vi "DIO_in.vi"(9 "Digital Pin":string(combo)="Y9", 11 "Data In":T1) -> (3 "Data Out":T1={"Port"="", "All Code"="Hi"})   [LabVIEW 2016]
uses:
  uPythonX/PythonData.ctl
  uPythonX/uPythonX.xctl
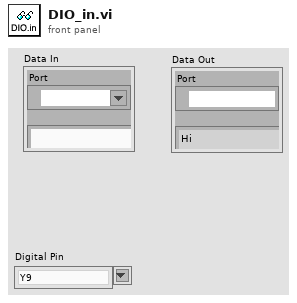
[diagram p1: front panel]
types:
  T1 = typedef "uPythonX.xctl/PythonData.ctl" = cluster{"Port":refnum<visa-resource-name>, "All Code":string}
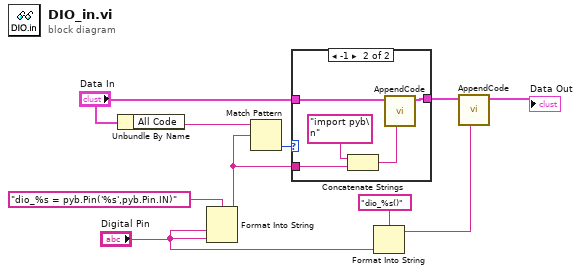
[diagram p0: block diagram]
diagram:
  n1 = Unbundle By Name("Data In") -> ("All Code"=w8:string)
  n2 = Format Into String(format string="dio_%s = pyb.Pin('%s',pyb.Pin.IN)", "Digital Pin", "Digital Pin") -> (resulting string=w5:string)  [unwired: 2 in, 1 out]
  n3 = Match Pattern(string=w8, regular expression=w5) -> (offset past match=w7:i32)  [unwired: 1 in, 3 out]
  n4 = case shown="-1" w7 {
    tunnel: "Data In" -> [w11 w16]
    tunnel: w5 -> [_ w13]
    tunnel: [w11 w15] -> w4
    frame Default {
    }
    frame -1 {
      n5 = Concatenate Strings("import pyb\n" ("format string"), w13) -> (w12:string)
      n6 = call "AppendCode.vi"("New Code"=w12, "Data In"=w16) -> ("Data Out"=w15:T1)  [unwired: 9 in]
    }
  }
  n7 = Format Into String(format string="dio_%s()", "Digital Pin") -> (resulting string=w1:string)  [unwired: 2 in, 1 out]
  n8 = call "AppendCode.vi"("New Code"=w1, "Data In"=w4) -> ("Data Out"=→"Data Out":T1)  [unwired: 9 in]
